vi "MSScript_SubVI_ArrayVarAccess.vi"(4 "Init Data":T1(array[cluster]), 5 "Function (Read)":enum16{"Init", "Write", "Read"}(ring)=enum."Read", 7 "ArrayVariable in":ext[](array[numeric]), 9 "VarName":string) -> (0 "Value Error?":bool, 1 "ArrayVariable out":ext[](array[numeric]), 2 "Is a variable ?":bool)   [LabVIEW 2018, in "MSScript.lvclass"]
uses:
  MSScript/MSScript.lvclass
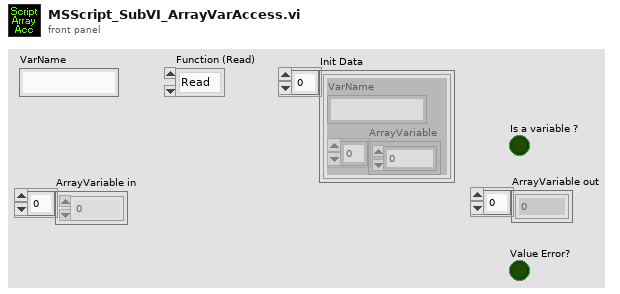
[diagram p1: front panel]
types:
  T1 = cluster{"VarName":string, "ArrayVariable":ext[]}[]
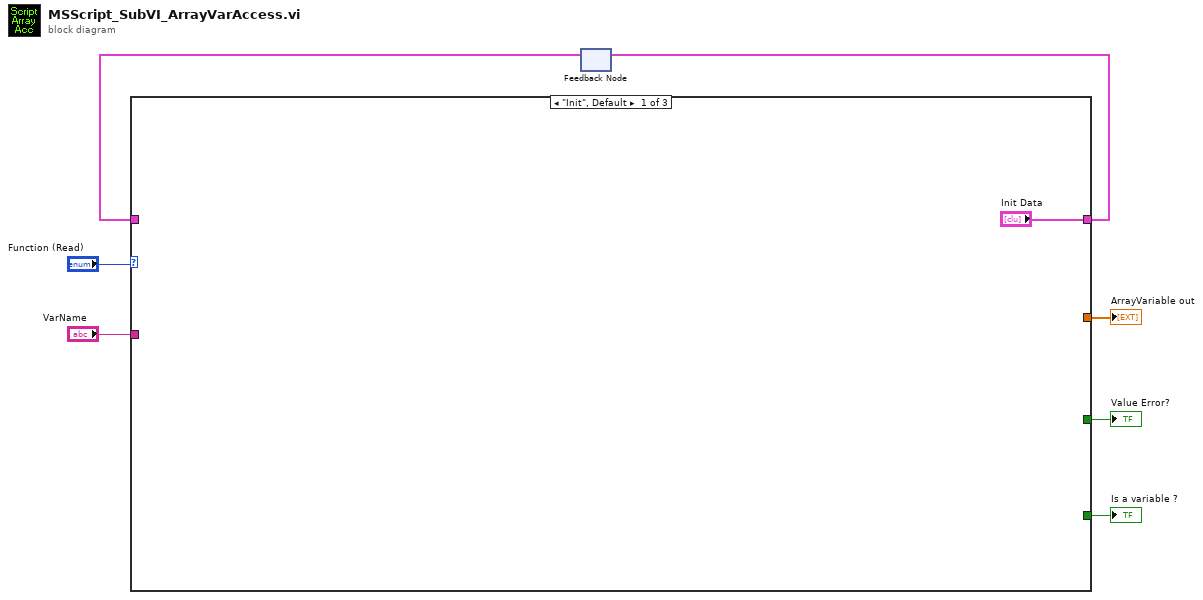
[diagram p0: block diagram]
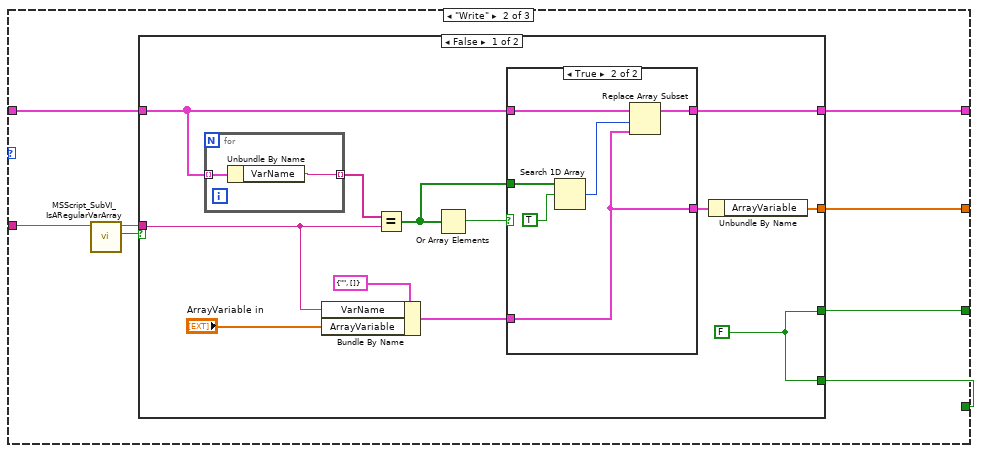
[diagram p2: hidden frame]
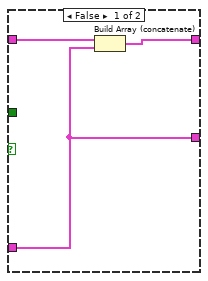
[diagram p3: hidden frame]
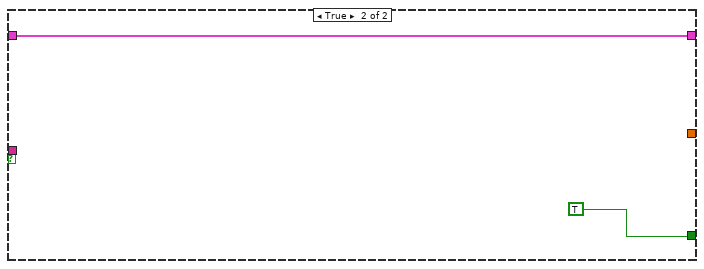
[diagram p4: hidden frame]
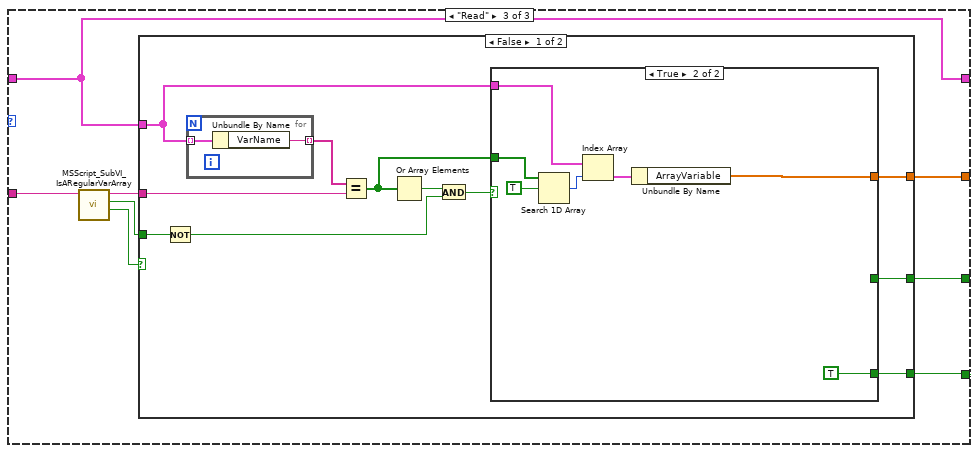
[diagram p5: hidden frame]
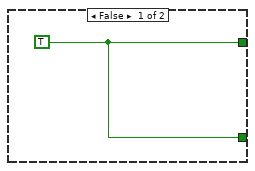
[diagram p6: hidden frame]
diagram:
  n1 = feedback #1() -> (w6:T1)  [unwired: 1 in]
  n2 = case shown="\"Init\", Default" "Function (Read)" {
    tunnel: ["Init Data" w15 w49] -> w5
    tunnel: w6 -> [_ w16 w49]
    tunnel: "VarName" -> [_ w11 w42]
    tunnel: [_ w14 w48] -> w3
    tunnel: [_ w13 w47] -> w2
    tunnel: [_ w12 w46] -> w1
    frame "Init", Default {
    }
    frame "Write" {
      n3 = call "MSScript_SubVI_IsARegularVarArray.vi"("VarString in"=w11) -> ("irregular"=w9:bool, "VarString out"=w10:string)  [unwired: 6 in, 1 out]
      n4 = case shown="False" w9 {
        tunnel: w16 -> [w26 w41]
        tunnel: [w23 w41] -> w15
        tunnel: [w22 _] -> w14
        tunnel: [w17 TRUE] -> w13
        tunnel: w10 -> [w21 _]
        tunnel: [w17 _] -> w12
        frame False {
          w17 = FALSE
          n5 = for {
            tunnel: w26 -> [w39] mode=indexing
            tunnel: [w38] -> w28 mode=indexing
            n6 = Unbundle By Name(w39) -> ("VarName"=w38:string)
          }
          n7 = Bundle By Name(cluster=cluster{"VarName":string, "ArrayVariable":ext[]} {"VarName"="", "ArrayVariable"=[]} ("VariableCluster"), "VarName"=w21, "ArrayVariable"="ArrayVariable in") -> (w25:cluster{"VarName":string, "ArrayVariable":ext[]})
          n8 = Equal?(x=w28, y=w21) -> (x = y?=w27:bool[])
          n9 = Or Array Elements(Boolean array=w27) -> (logical OR=w20:bool)
          n10 = case shown="True" w20 {
            tunnel: w27 -> [_ w37]
            tunnel: w26 -> [w31 w33]
            tunnel: w25 -> [w29 w32]
            tunnel: [w30 w34] -> w23
            tunnel: [w29 w32] -> w24
            frame False {
              n11 = Build Array (concatenate)(w31, w29) -> (w30:T1)
            }
            frame True {
              n12 = Search 1D Array(1D array=w37, element=TRUE) -> (index of element=w35:i32)  [unwired: 1 in]
              n13 = Replace Array Subset(array=w33, new element=w32, index=w35) -> (w34:T1)
            }
          }
          n14 = Unbundle By Name(w24) -> ("ArrayVariable"=w22:ext[])
        }
        frame True {
        }
      }
    }
    frame "Read" {
      n15 = call "MSScript_SubVI_IsARegularVarArray.vi"("VarString in"=w42) -> ("Variable simbol no found"=w44:bool, "irregular"=w43:bool, "VarString out"=w45:string)  [unwired: 6 in]
      n16 = case shown="False" w44 {
        tunnel: w45 -> [w50 _]
        tunnel: w49 -> [w57 _]
        tunnel: [w56 _] -> w48
        tunnel: [w52 _] -> w47
        tunnel: [w51 _] -> w46
        tunnel: w43 -> [w53 _]
        frame False {
          n17 = Not(x=w53) -> (.not. x?=w55:bool)
          n18 = for {
            tunnel: [w70] -> w60 mode=indexing
            tunnel: w57 -> [w69] mode=indexing
            n19 = Unbundle By Name(w69) -> ("VarName"=w70:string)
          }
          n20 = Equal?(x=w60, y=w50) -> (x = y?=w58:bool[])
          n21 = Or Array Elements(Boolean array=w58) -> (logical OR=w59:bool)
          n22 = And(x=w59, y=w55) -> (x .and. y?=w54:bool)
          n23 = case shown="True" w54 {
            tunnel: w58 -> [_ w68]
            tunnel: w57 -> [_ w66]
            tunnel: [_ w62] -> w56
            tunnel: [w61 _] -> w52
            tunnel: [w61 TRUE] -> w51
            frame False {
              w61 = TRUE
            }
            frame True {
              n24 = Search 1D Array(1D array=w68, element=TRUE) -> (index of element=w65:i32)  [unwired: 1 in]
              n25 = Index Array(array=w66, index=w65) -> (element=w64:cluster{"VarName":string, "ArrayVariable":ext[]})
              n26 = Unbundle By Name(w64) -> ("ArrayVariable"=w62:ext[])
            }
          }
        }
        frame True {
        }
      }
    }
  }
  "ArrayVariable out" <- w3
  "Is a variable ?" <- w1
  "Value Error?" <- w2
  n27 = feedback-in #1(w5) -> ()
